vi "MathFinder_Case-Plus-Mul.vi"(0 "Whole Match":string, 7 "After Match":string, 11 "error in (no error)":errorcluster) -> (4 "in1":string, 6 "Expression":string, 8 "in2":string, 15 "error out":errorcluster {"code" format="%f"})   [LabVIEW 2014]
uses:
  <vilib>/regexp/Match Regular Expression.xnode
panel:
  out "Intermediate String":string
  out "Empty String":string
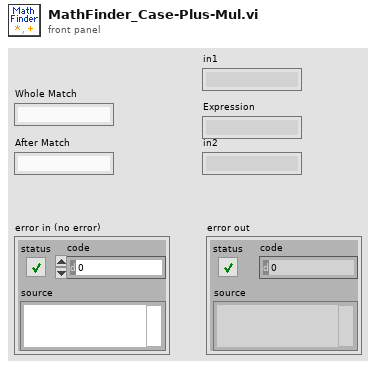
[diagram p1: front panel]
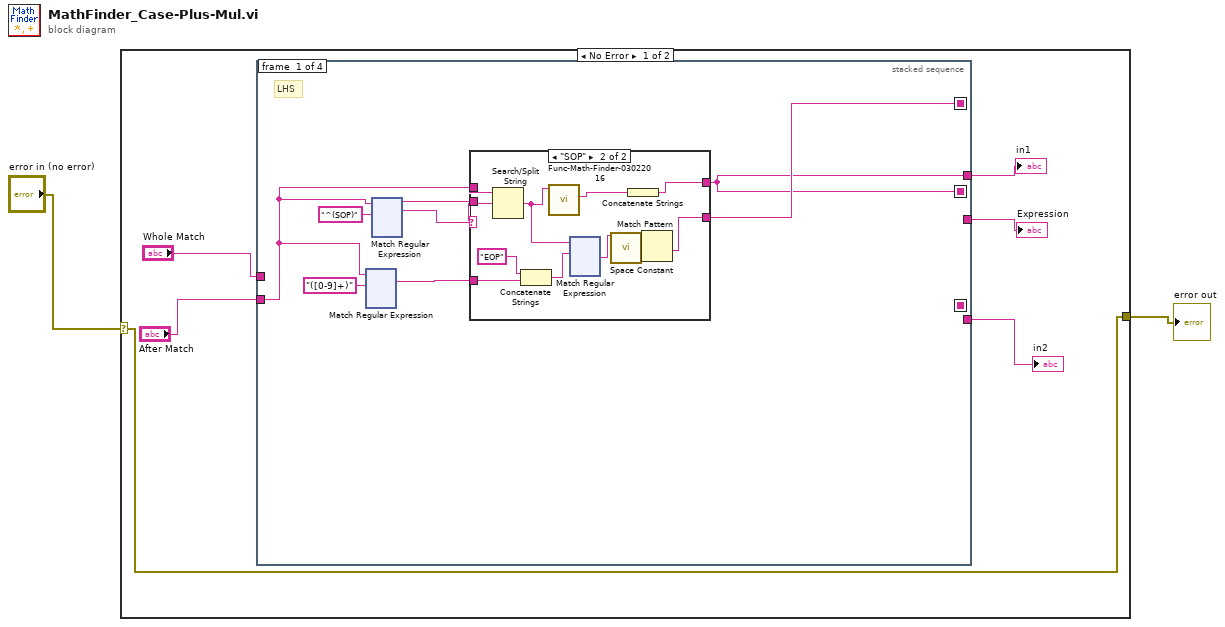
[diagram p0: block diagram]
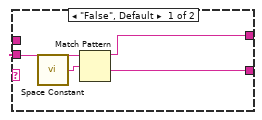
[diagram p2: hidden frame]
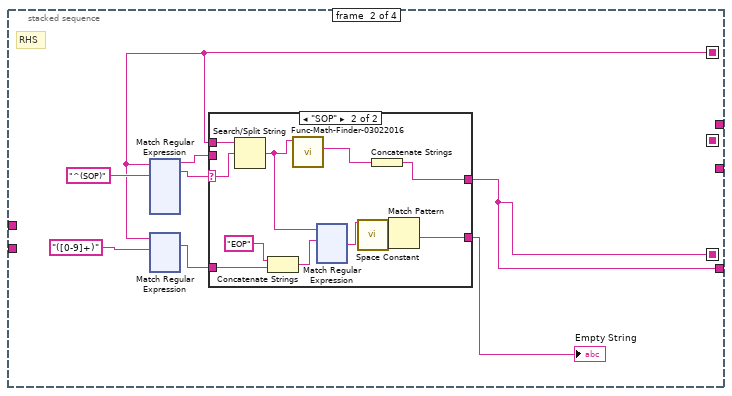
[diagram p3: hidden frame]
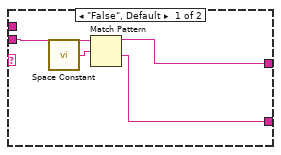
[diagram p4: hidden frame]
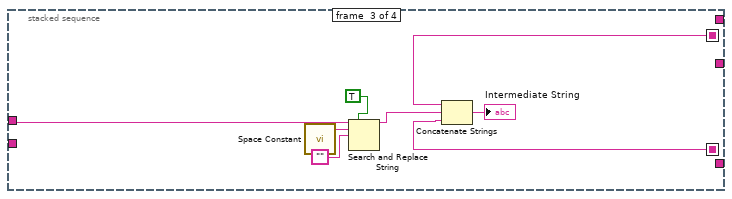
[diagram p5: hidden frame]
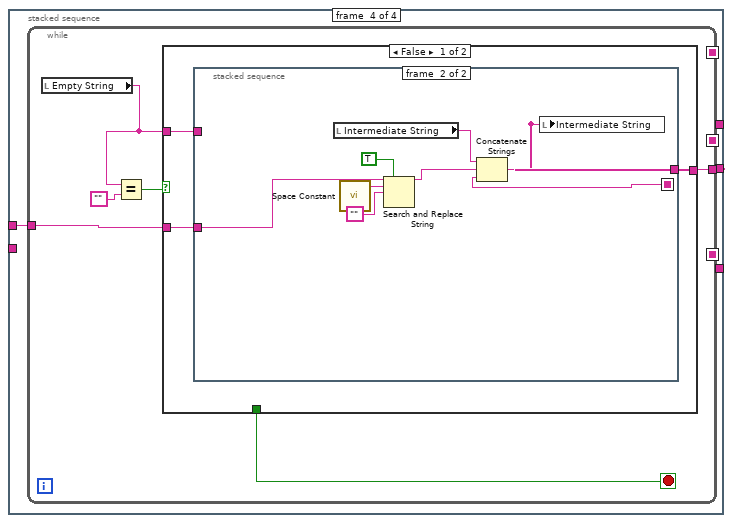
[diagram p6: hidden frame]
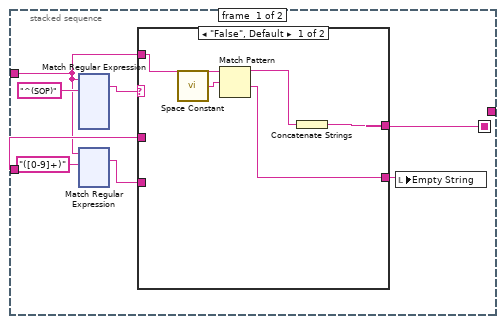
[diagram p7: hidden frame]
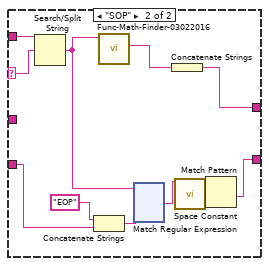
[diagram p8: hidden frame]
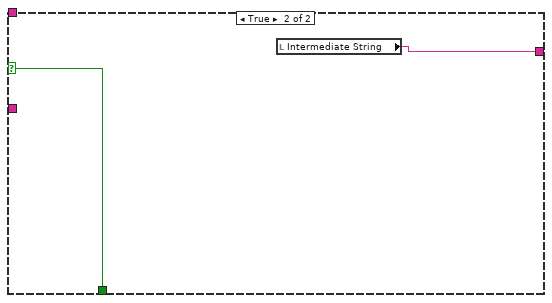
[diagram p9: hidden frame]
diagram:
  n1 = case shown="No Error" "error in (no error)" {
    selector: "error in (no error)" -> [w3 w1140]
    tunnel: [w3 w1140] -> w1
    frame No Error {
      n2 = stacked-sequence {
        seq-local: [w14 _ _ _] -> [_ w376 _ _]
        seq-local: [_ w378 _ _] -> [_ _ w743 _]
        seq-local: [w13 _ _ _] -> [_ _ w744 _]
        tunnel: "After Match" -> [w9 _ _ _]
        tunnel: "Whole Match" -> [_ _ w745 w750]
        tunnel: [_ w378 _ _] -> w5
        tunnel: [w13 _ _ _] -> w6
        tunnel: [_ _ _ w751] -> w4
        frame #0 {
          # "LHS"
          n3 = xnode "Match Regular Expression"("input string"=w9, "regular expression"="([0-9]+)") -> ("whole match"=w10:string)  [unwired: 4 in, 4 out]
          n4 = xnode "Match Regular Expression"("input string"=w9, "regular expression"="^(SOP)") -> ("before match"=w15:string, "whole match"=w12:string)  [unwired: 4 in, 3 out]
          n5 = case shown="\"SOP\"" w12 {
            selector: w12 -> [_ w144]
            tunnel: w15 -> [w134 _]
            tunnel: [w132 w137] -> w14
            tunnel: [w131 w135] -> w13
            tunnel: w9 -> [_ w145]
            tunnel: w10 -> [_ w142]
            frame "False", Default {
              n6 = call <vilib>:"Space Constant.vi"() -> ("String"=w133:string)
              n7 = Match Pattern(string=w134, regular expression=w133) -> (before substring=w131:string, after substring=w132:string)  [unwired: 1 in, 2 out]
            }
            frame "SOP" {
              n8 = Search/Split String(string=w145, search string/char (-)=w144) -> (match + rest of string=w140:string)  [unwired: 1 in, 2 out]
              n9 = Concatenate Strings("EOP" ("regular expression"), w142) -> (w141:string)
              n10 = call "Func-Math-Finder-03022016.vi"("Get Tagged String"=w140) -> ("Expression"=w136:string)  [unwired: 8 in, 2 out]
              n11 = xnode "Match Regular Expression"("input string"=w140, "regular expression"=w141) -> ("after match"=w138:string)  [unwired: 4 in, 4 out]
              n12 = call <vilib>:"Space Constant.vi"() -> ("String"=w139:string)
              n13 = Concatenate Strings(w136) -> (w135:string)
              n14 = Match Pattern(string=w138, regular expression=w139) -> (after substring=w137:string)  [unwired: 1 in, 3 out]
            }
          }
        }
        frame #1 {
          # "RHS"
          n15 = xnode "Match Regular Expression"("input string"=w376, "regular expression"="^(SOP)") -> ("before match"=w379:string, "whole match"=w380:string)  [unwired: 4 in, 5 out]
          n16 = xnode "Match Regular Expression"("input string"=w376, "regular expression"="([0-9]+)") -> ("whole match"=w375:string)  [unwired: 4 in, 4 out]
          n17 = case shown="\"SOP\"" w380 {
            selector: w380 -> [_ w509]
            tunnel: w379 -> [w499 _]
            tunnel: [w497 w508] -> w378
            tunnel: w376 -> [_ w510]
            tunnel: w375 -> [_ w502]
            tunnel: [w496 w500] -> w374
            frame "False", Default {
              n18 = call <vilib>:"Space Constant.vi"() -> ("String"=w498:string)
              n19 = Match Pattern(string=w499, regular expression=w498) -> (before substring=w497:string, after substring=w496:string)  [unwired: 1 in, 2 out]
            }
            frame "SOP" {
              n20 = Search/Split String(string=w510, search string/char (-)=w509) -> (match + rest of string=w501:string)  [unwired: 1 in, 2 out]
              n21 = Concatenate Strings("EOP" ("regular expression"), w502) -> (w504:string)
              n22 = call "Func-Math-Finder-03022016.vi"("Get Tagged String"=w501) -> ("Expression"=w507:string)  [unwired: 8 in, 2 out]
              n23 = xnode "Match Regular Expression"("input string"=w501, "regular expression"=w504) -> ("after match"=w506:string)  [unwired: 4 in, 4 out]
              n24 = call <vilib>:"Space Constant.vi"() -> ("String"=w503:string)
              n25 = Concatenate Strings(w507) -> (w508:string)
              n26 = Match Pattern(string=w506, regular expression=w503) -> (after substring=w500:string)  [unwired: 1 in, 3 out]
            }
          }
          "Empty String" <- w374
        }
        frame #2 {
          n27 = call <vilib>:"Space Constant.vi"() -> ("String"=w748:string)
          n28 = Search and Replace String(replace all?=TRUE ("replace all? (F)"), input string=w745, search string=w748, replace string="" ("string")) -> (result string=w746:string)  [unwired: 4 in, 3 out]
          n29 = Concatenate Strings(w744, w746, w743) -> (→"Intermediate String":string)
        }
        frame #3 {
          n30 = while {
            tunnel: [w755] -> w751
            tunnel: w750 -> [w754]
            stop <- w753 stop-if-true
            n31 = local read "Empty String"() -> (w752:string)
            n32 = Equal?(x=w752, y="") -> (x = y?=w756:bool)
            n33 = case shown="False" w756 {
              selector: w756 -> [_ w1139]
              tunnel: [w759 w1138] -> w755
              tunnel: w754 -> [w760 _]
              tunnel: [_ w1139] -> w753
              tunnel: w752 -> [w758 _]
              frame False {
                n34 = stacked-sequence {
                  seq-local: [w764 _] -> [_ w1132]
                  tunnel: w760 -> [w763 w1133]
                  tunnel: [_ w1130] -> w759
                  tunnel: w758 -> [w762 _]
                  frame #0 {
                    n35 = xnode "Match Regular Expression"("input string"=w762, "regular expression"="^(SOP)") -> ("whole match"=w767:string)  [unwired: 4 in, 6 out]
                    n36 = xnode "Match Regular Expression"("input string"=w762, "regular expression"="([0-9]+)") -> ("whole match"=w765:string)  [unwired: 4 in, 4 out]
                    n37 = case shown="\"False\", Default" w767 {
                      selector: w767 -> [_ w898]
                      tunnel: w762 -> [w887 w889]
                      tunnel: w765 -> [_ w893]
                      tunnel: [w885 w891] -> w761
                      tunnel: [w884 w890] -> w764
                      tunnel: w763 -> [_ _]
                      frame "False", Default {
                        n38 = call <vilib>:"Space Constant.vi"() -> ("String"=w886:string)
                        n39 = Match Pattern(string=w887, regular expression=w886) -> (before substring=w883:string, after substring=w885:string)  [unwired: 1 in, 2 out]
                        n40 = Concatenate Strings(w883) -> (w884:string)
                      }
                      frame "SOP" {
                        n41 = Search/Split String(string=w889, search string/char (-)=w898) -> (match + rest of string=w892:string)  [unwired: 1 in, 2 out]
                        n42 = Concatenate Strings("EOP" ("regular expression"), w893) -> (w895:string)
                        n43 = call "Func-Math-Finder-03022016.vi"("Get Tagged String"=w892) -> ("Expression"=w888:string)  [unwired: 8 in, 2 out]
                        n44 = xnode "Match Regular Expression"("input string"=w892, "regular expression"=w895) -> ("after match"=w897:string)  [unwired: 4 in, 4 out]
                        n45 = Concatenate Strings(w888) -> (w890:string)
                        n46 = call <vilib>:"Space Constant.vi"() -> ("String"=w894:string)
                        n47 = Match Pattern(string=w897, regular expression=w894) -> (after substring=w891:string)  [unwired: 1 in, 3 out]
                      }
                    }
                    n48 = local write "Empty String"(w761) -> ()
                  }
                  frame #1 {
                    n49 = local read "Intermediate String"() -> (w1131:string)
                    n50 = call <vilib>:"Space Constant.vi"() -> ("String"=w1136:string)
                    n51 = Search and Replace String(replace all?=TRUE ("replace all? (F)"), input string=w1133, search string=w1136, replace string="" ("string")) -> (result string=w1134:string)  [unwired: 4 in, 3 out]
                    n52 = Concatenate Strings(w1131, w1134, w1132) -> (w1130:string)
                    n53 = local write "Intermediate String"(w1130) -> ()
                  }
                }
              }
              frame True {
                n54 = local read "Intermediate String"() -> (w1138:string)
              }
            }
          }
        }
      }
      "in1" <- w6
      "in2" <- w5
      "Expression" <- w4
    }
    frame Error {
    }
  }
  "error out" <- w1
